vi "ConvertTbl2ChanGrp.vi"(8 "error in (no error)":errorcluster, 9 "ItemNames":string[][](array[string]), 10 "ge_DAQManDefinitions":T1, 11 "ChanGrp in":refnum<class "ChanGrp.lvclass">) -> (0 "error out":errorcluster, 3 "ChanGrp in":refnum<class "ChanGrp.lvclass">)   [LabVIEW 2012, in "Configuration Grandmaster.lvlib" / "ChanGrp.lvclass"]
uses:
  ChanGrp.lvclass
  Common/Controls/DAQMan Definitions.ctl
  ChanGrp.lvclass/ChanGrp.ctl
  Read MeasType.vi
  Measurements/Class Channel/Channel.lvclass
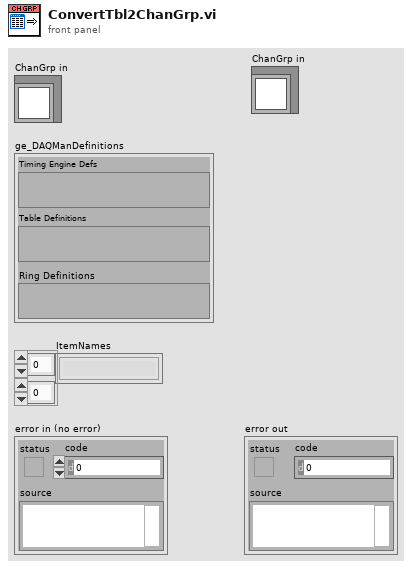
[diagram p1: front panel]
types:
  T1 = typedef "DAQMan Definitions.ctl" = cluster{"Timing Engine Defs":variant, "Table Definitions":variant, "Ring Definitions":variant}
  T2 = typedef "ge_MeasType.ctl" = enum16{"Voltage", "Frequency", "Tachometer", "Dynamic", "Thermocouple", "RTD", "Strain", "Current", "Resistance"}
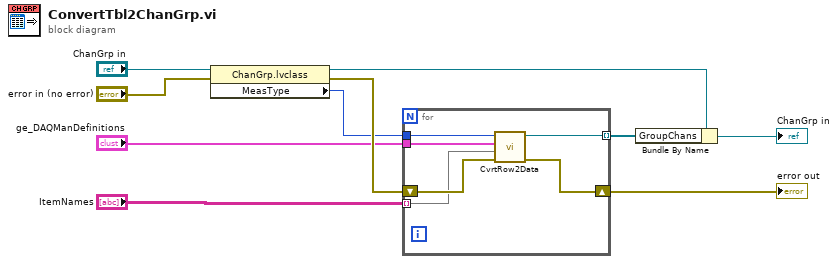
[diagram p0: block diagram]
diagram:
  n1 = property class="ChanGrp.lvclass"(reference="ChanGrp in", error in="error in (no error)") -> (reference out=w8:refnum<class "ChanGrp.lvclass">, error out=w10:errorcluster, "MeasType"=w5:T2)
  n2 = for {
    tunnel: "ItemNames" -> [w12] mode=indexing
    tunnel: w5 -> [w11]
    tunnel: [w16] -> w3 mode=indexing
    shift-right: [w14] -> w1
    shift-left: w10 -> [w15]
    tunnel: "ge_DAQManDefinitions" -> [w13]
    n3 = call "CvrtRow2Data.vi"("error in (no error)"=w15, "Item Names"=w12, "ge_DAQManDefinitions"=w13, "MeasType"=w11) -> ("error out"=w14:errorcluster, "Channel out"=w16:refnum<class "Channel.lvclass">)  [unwired: 6 in]
  }
  "error out" <- w1
  n4 = Bundle By Name(cluster=w8, "GroupChans"=w3) -> (→"ChanGrp in":refnum<class "ChanGrp.lvclass">)
